vi "Pack Message.vi"(8 "error in (no error)":errorcluster, 11 "Message Response in":refnum<class "Message Response.lvclass">) -> (0 "error out":errorcluster, 1 "Packed Message":string, 2 "Message Name":string, 3 "Message Response out":refnum<class "Message Response.lvclass">)   [LabVIEW 2016, in "WebSocket Networking.lvlib" / "Message Response.lvclass"]
uses:
  <userlib>/Common Components/WebSocket Networking/Message Response/Message Response.lvclass
  C:/Program Files (x86)/National Instruments/LabVIEW 2016/user.lib/Composed Systems/Stream/Mediator/Classes/Message Interface/Message Interface.lvclass
  <userlib>/Common Components/WebSocket Networking/Message Response/Message Response.lvclass/Message Response.ctl
  <userlib>/Composed Systems/Stream/Mediator/Classes/Message Interface/Message Interface.lvclass
  <vilib>/addons/_JKI.lib/Serialization/JSON/JKI JSON Serialization.lvlib
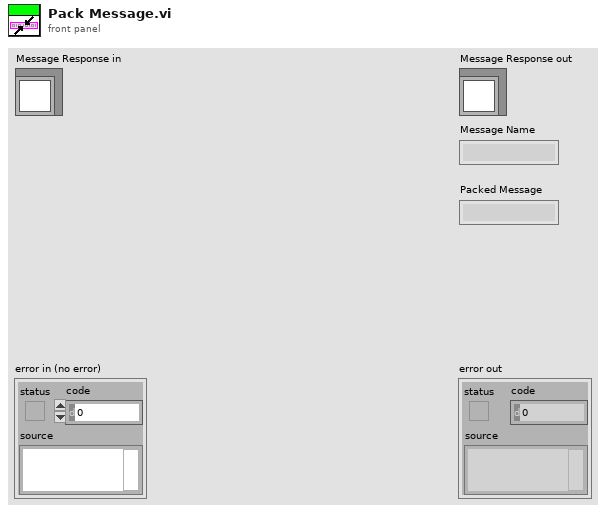
[diagram p1: front panel]
types:
  T1 = typedef "Common.lvlib/command-data.ctl" = cluster{"command":string, "data":string}
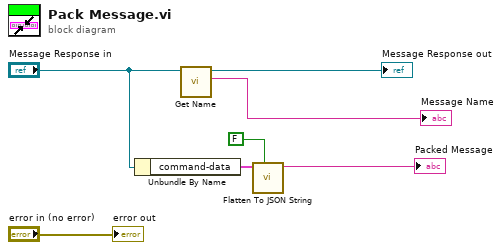
[diagram p0: block diagram]
diagram:
  n1 = Unbundle By Name("Message Response in") -> ("command-data"=w3:T1)
  n2 = call <userlib>:"Get Name.vi"("Message Interface in"="Message Response in") -> ("Name"=→"Message Name":string, "Message Interface out"=→"Message Response out":refnum<class "Message Response.lvclass">)  [unwired: 8 in, 1 out]
  n3 = call <vilib>:"Flatten To JSON String.vi"("Multiline (T)"=FALSE, "Variant"=w3) -> ("JSON String"=→"Packed Message":string)  [unwired: 8 in, 1 out]
  "error out" <- "error in (no error)"
